vi "Screw Print.vi"(8 "error in (no error)":errorcluster, 10 "On?":bool, 11 "Feeder Actor.lvlib:Screw in":refnum<class "Screw.lvclass">) -> (0 "error out":errorcluster, 3 "Feeder Actor.lvlib:Screw out":refnum<class "Screw.lvclass">)   [LabVIEW 2018, in "Feeder Actor.lvlib" / "Screw.lvclass"]
uses:
  Screw.lvclass
  C:/Program Files/National Instruments/LabVIEW 2018/vi.lib/ActorFramework/Actor/Actor.lvclass
  <vilib>/ActorFramework/Actor/Actor.lvclass/Actor.ctl
  <vilib>/ActorFramework/Message Enqueuer/Message Enqueuer.lvclass/Message Enqueuer.ctl
  Screw.lvclass/Screw.ctl
  <vilib>/ActorFramework/Message Enqueuer/Init from Existing Queue.vi
  <vilib>/ActorFramework/Message Enqueuer/Message Enqueuer.lvclass
  <vilib>/ActorFramework/Actor/Actor.lvclass
  Screw Messages/Set Screw Msg/Set Screw Msg.lvclass
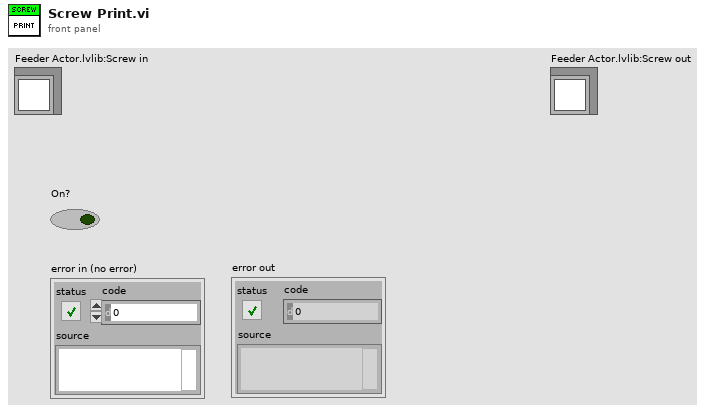
[diagram p1: front panel]
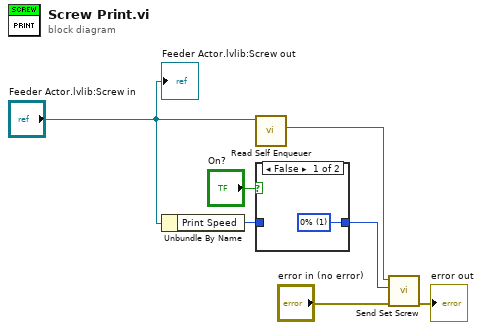
[diagram p0: block diagram]
diagram:
  n1 = Unbundle By Name("Feeder Actor.lvlib:Screw in") -> ("Print Speed"=w6:u16)
  n2 = call <vilib>:"Read Self Enqueuer.vi"("Actor"="Feeder Actor.lvlib:Screw in") -> ("Self Enqueuer"=w7:refnum<class "Message Enqueuer.lvclass">)  [unwired: 10 in]
  n3 = case shown="False" "On?" {
    tunnel: w6 -> [_ w9]
    tunnel: [w8 w9] -> w2
    frame False {
      w8 = u16 1 items=["0%"=1, "25%"=225, "50%"=450, "75%"=675, "100%"=900] ("Screw")
    }
    frame True {
    }
  }
  n4 = call "Send Set Screw.vi"("error in (no error)"="error in (no error)", "Screw"=w2, "Message Enqueuer in"=w7) -> ("error out"=→"error out":errorcluster)  [unwired: 7 in, 1 out]
  "Feeder Actor.lvlib:Screw out" <- "Feeder Actor.lvlib:Screw in"
